vi "Split Address Range.vi"(9 "max number of items":u16, 10 "number of items":u16, 11 "address":u16) -> (3 "addresses and numbers of items":cluster{"address":u16, "number of items":u16}[](array[cluster]))   [LabVIEW 2020, in "Library Instrument & Equipement.lvlib" / "Library Relay_Board.lvlib" / "Modbus.lvclass"]
doc: "Splits single address range specified by <B>address</B> and <B>number of items</B> into number of ranges with size limited by <B>max number of items</B>."
uses:
  Modbus.lvclass
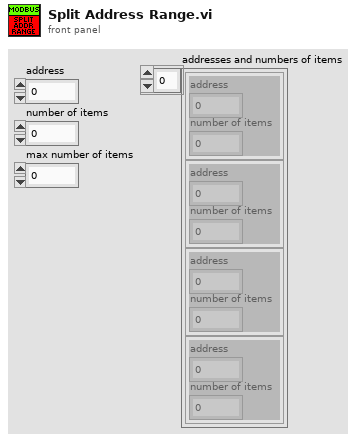
[diagram p1: front panel]
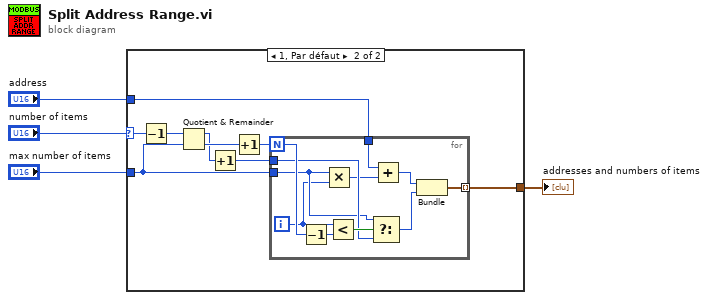
[diagram p0: block diagram]
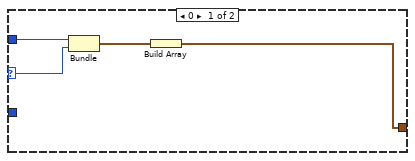
[diagram p2: hidden frame]
diagram:
  n1 = case shown="1, Par défaut" "number of items" {
    selector: "number of items" -> [w7 w11]
    tunnel: "address" -> [w8 w15]
    tunnel: "max number of items" -> [_ w14]
    tunnel: [w5 w13] -> w2
    frame 0 {
      n2 = Bundle("address"=w8, "number of items"=w7) -> (w6:cluster{"address":u16, "number of items":u16})  [unwired: 1 in]
      n3 = Build Array(w6) -> (w5:cluster{"address":u16, "number of items":u16}[])
    }
    frame 1, Default {
      n4 = Decrement(x=w11) -> (x-1=w12:u16)
      n5 = Quotient & Remainder(x=w12, y=w14) -> (x-y*floor(x/y)=w10:u16, floor(x/y)=w17:u16)
      n6 = Increment(x=w10) -> (x+1=w9:u16)
      n7 = Increment(x=w17) -> (x+1=w16:u16)
      n8 = for {
        N: w16 -> [w25]
        tunnel: w15 -> [w28]
        tunnel: w14 -> [w19]
        tunnel: [w26] -> w13 mode=indexing
        tunnel: w9 -> [w22]
        i -> [w18]
        n9 = Decrement(x=w25) -> (x-1=w24:i32)
        n10 = Multiply(x=w19, y=w18) -> (x*y=w20:i32)
        n11 = Less?(x=w18, y=w24) -> (x < y?=w23:bool)
        n12 = Select(t=w19, s=w23, f=w22) -> (s? t:f=w21:u16)
        n13 = Add(x=w28, y=w20) -> (x+y=w27:i32)
        n14 = Bundle(w27, "max number of items"=w21) -> (w26:cluster{i32, "max number of items":u16})  [unwired: 1 in]
      }
    }
  }
  "addresses and numbers of items" <- w2
